vi "Electrolytic Separater.vi"(4 "Speed Upgrades":u32 max=8) -> (2 "Hydrogen (mB/t)":u32, 3 "Oxygen (mB/t)":u32)   [LabVIEW 2023]
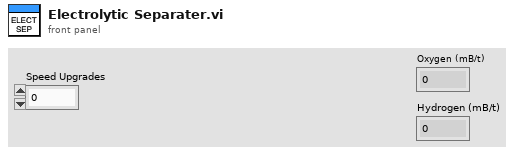
[diagram p1: front panel]
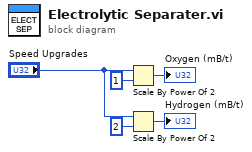
[diagram p0: block diagram]
diagram:
  n1 = Scale By Power Of 2(n="Speed Upgrades", x=u32 1) -> (x*2^n=→"Oxygen (mB/t)":u32)
  n2 = Scale By Power Of 2(n="Speed Upgrades", x=u32 2) -> (x*2^n=→"Hydrogen (mB/t)":u32)
